vi "MB_TCP_7024_p.vi"(6 "N":i32, 9 "timeouts":T1={"conn_timeout"=1000, "reconn_timeout"=3000, "N attempt max"=3, "t_reset_TTL"=120000, "write_timeout"=10, "read_timeout"=500, "period"=100} {"t_reset_TTL" min=10 max=240000 step=1; "period" min=10 max=100000 step=1; "read_timeout" min=10 max=60000 step=1; "write_timeout" min=1 max=60000 step=1; "N attempt max" min=1 max=5 step=1; "reconn_timeout" min=10 max=240000 step=1; "conn_timeout" min=10 max=240000}, 10 "write enable":bool=TRUE, 11 "stop":bool) -> (0 "error out":errorcluster, 2 "errors":u32, 3 "Z3":u32)   [LabVIEW 2019]
uses:
  NI_modbus_upd/NI_modbus_upd.lvlib
  NI_modbus_upd.llb/MB Modbus Command.ctl
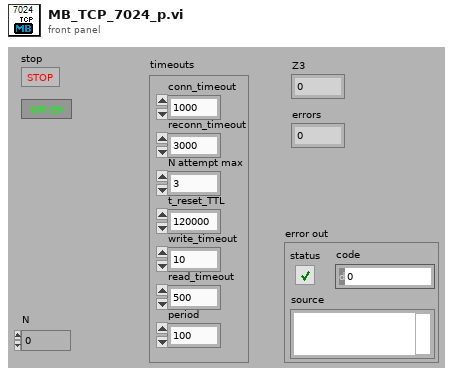
[diagram p1: front panel]
types:
  T1 = cluster{"conn_timeout":i32, "reconn_timeout":u32, "N attempt max":i32, "t_reset_TTL":u32, "write_timeout":i32, "read_timeout":i32, "period":u32}
  T2 = enum16{"Init", "Read", "Read inputs", "Read outputs", "Write", "Write inputs"}
  T3 = enum16{"DI", "DO to write", "DO", "AI", "AO to write", "AO", "DI AI", "DI AO", "DO AI", "DO AO"}
  T4 = enum16{"Start", "Connect", "Write enable", "IP address", "Errors"}
  T5 = typedef "MB Modbus Command.ctl" = cluster{"Function Code":u8, "Starting Address":u16, "Quantity":u16, "Data":u16[], "Discrete":bool[]}
  T6 = cluster{"Transaction ID":u16, "Protocol ID":u16, "Length":u16, "Unit ID":u8}
  T7 = cluster{"Remote IP Address":string, "Remote Port":u16}
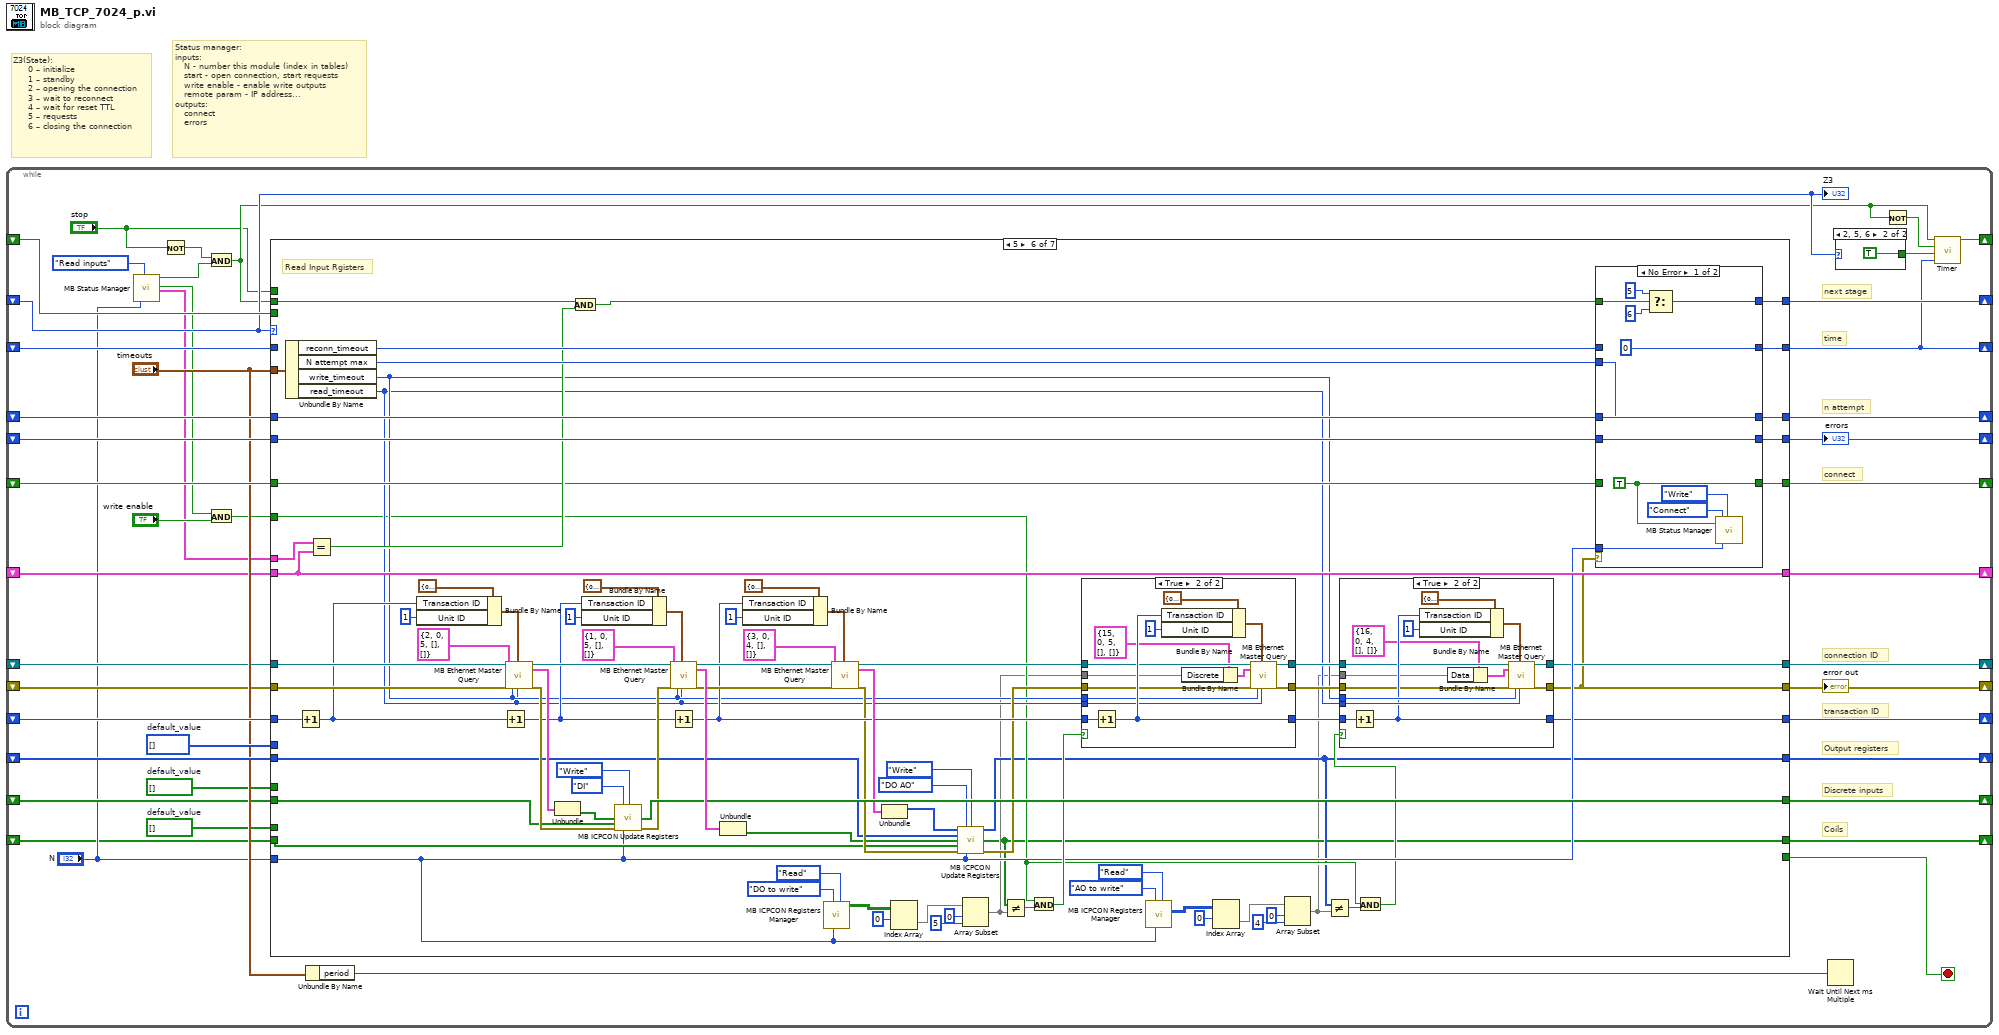
[diagram p0: block diagram]
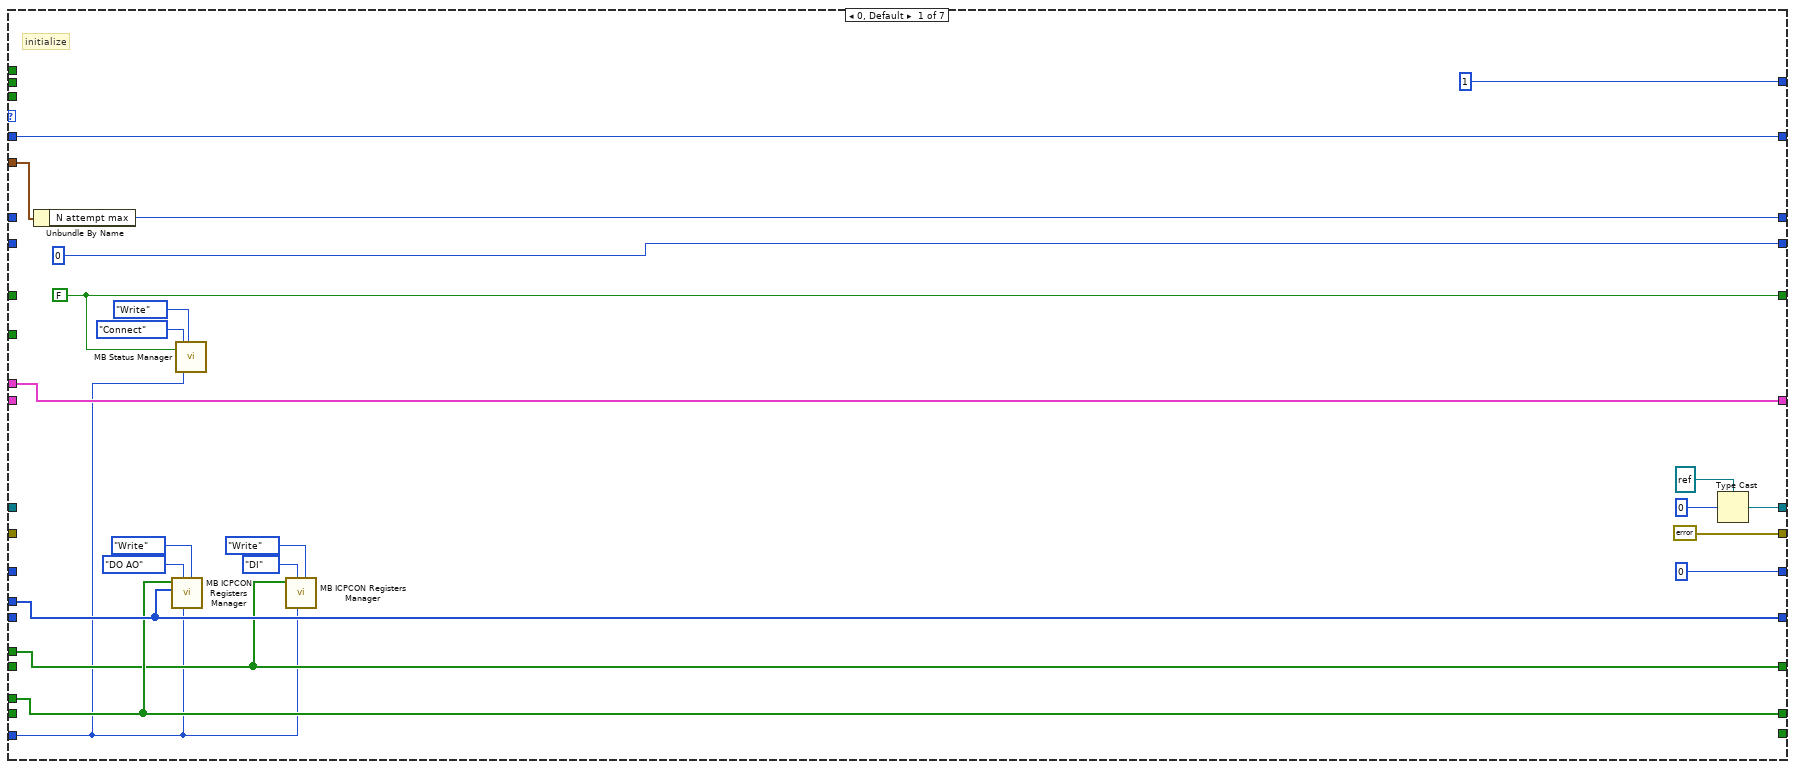
[diagram p2: hidden frame]
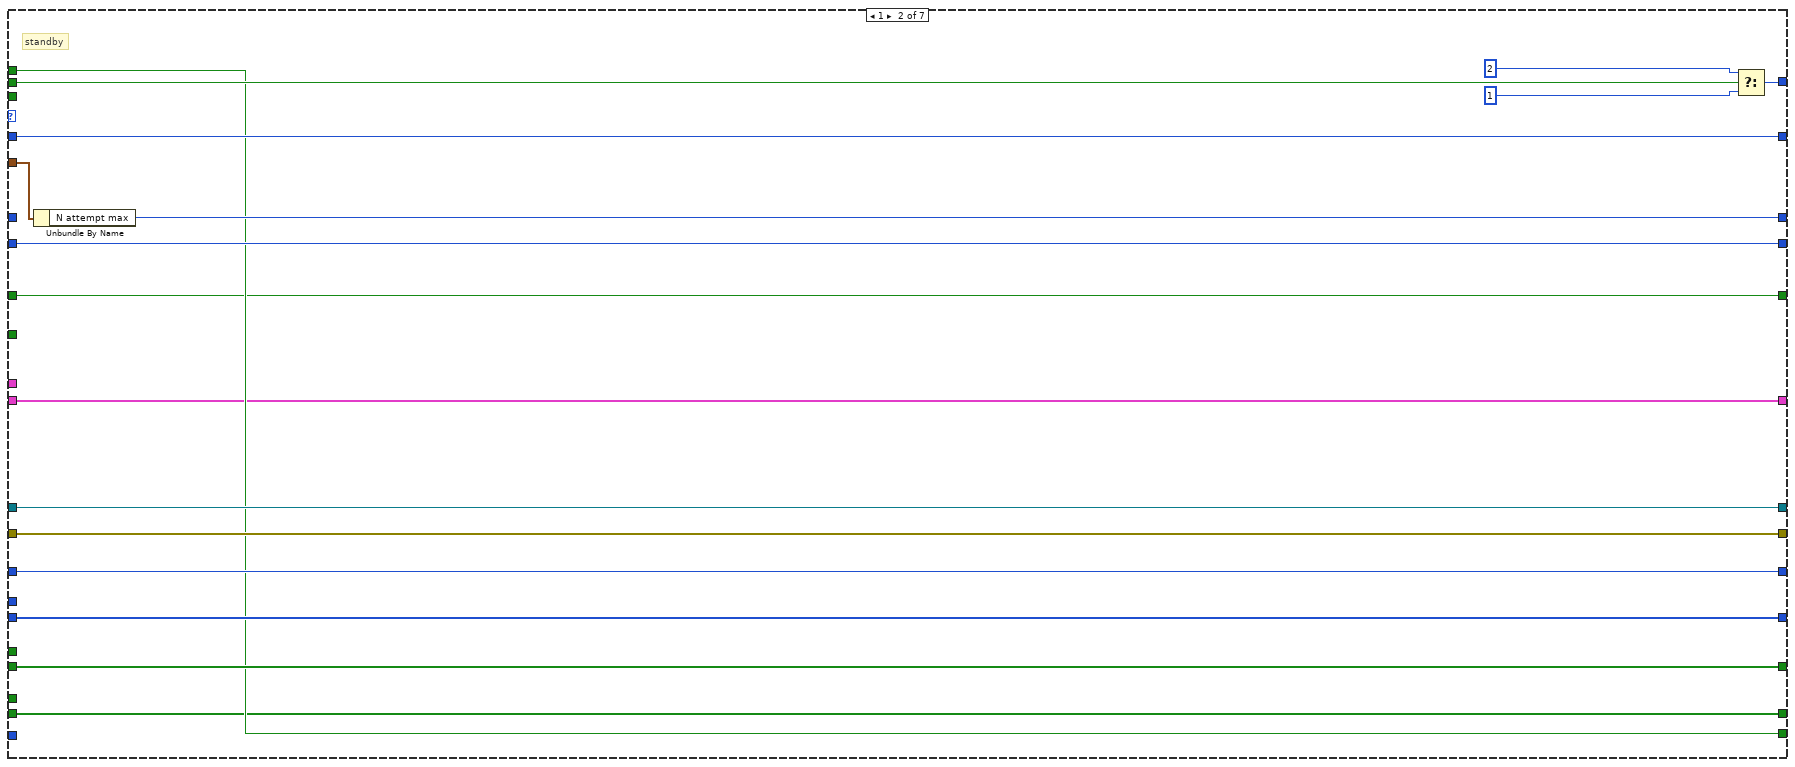
[diagram p3: hidden frame]
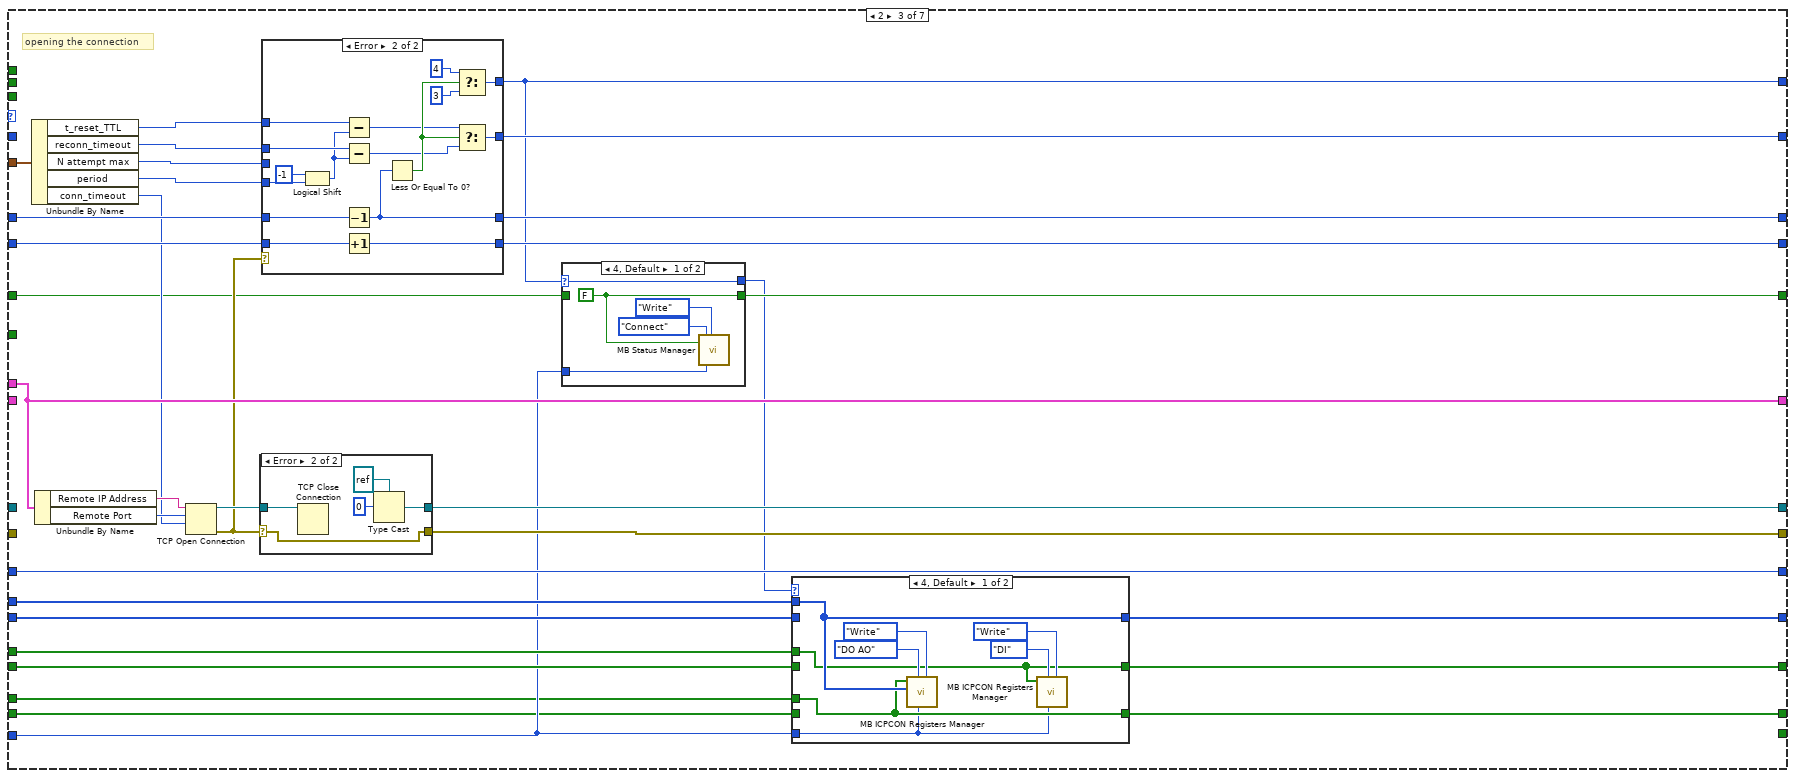
[diagram p4: hidden frame]
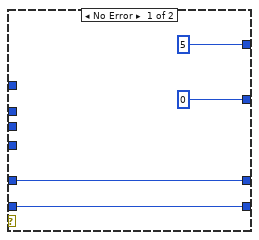
[diagram p8: hidden frame]
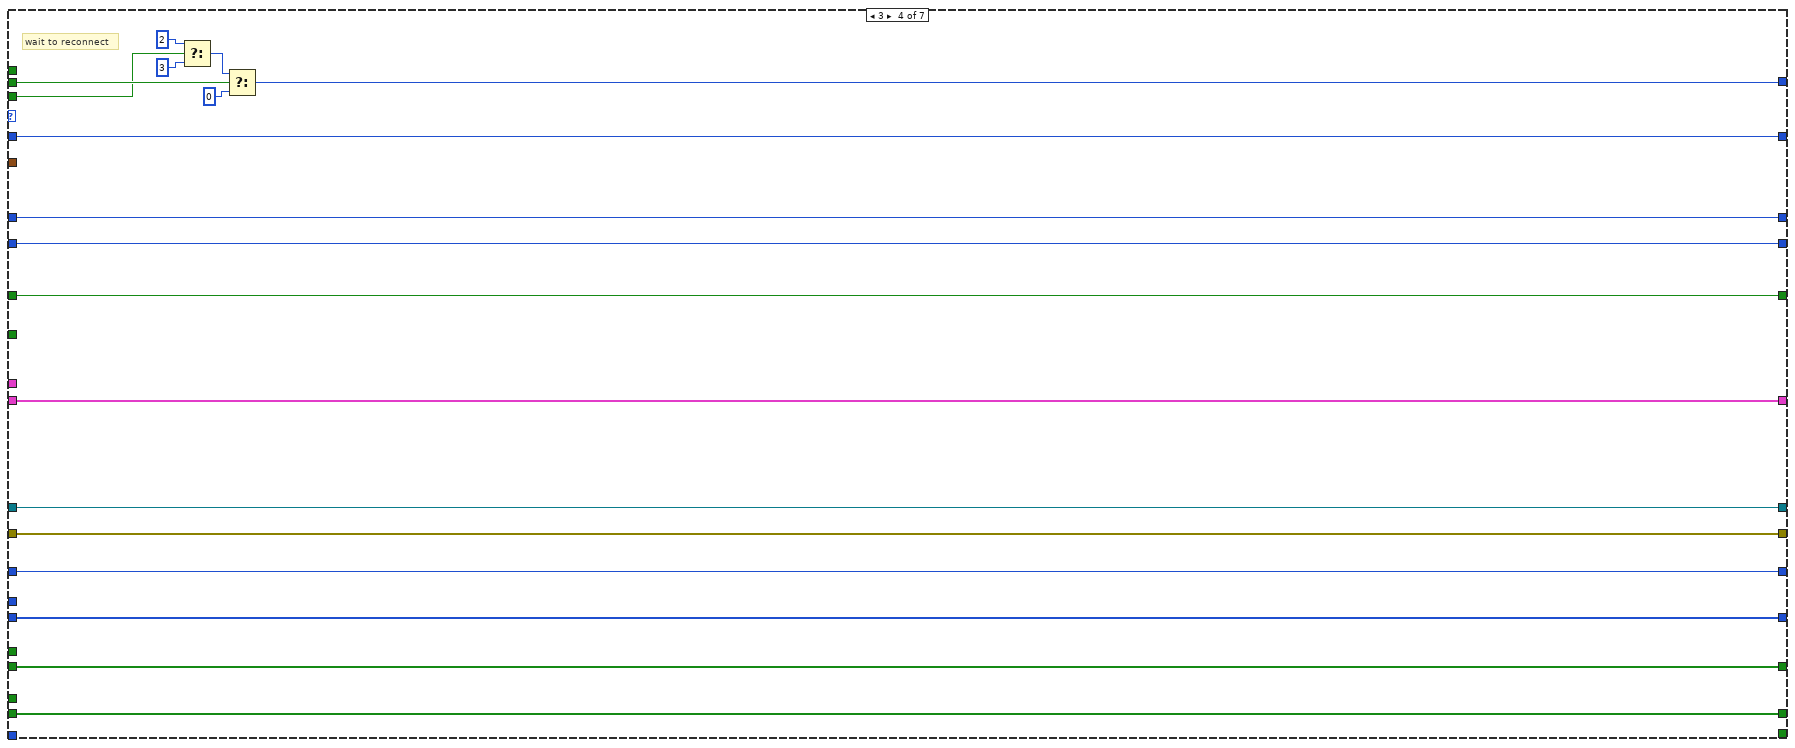
[diagram p9: hidden frame]
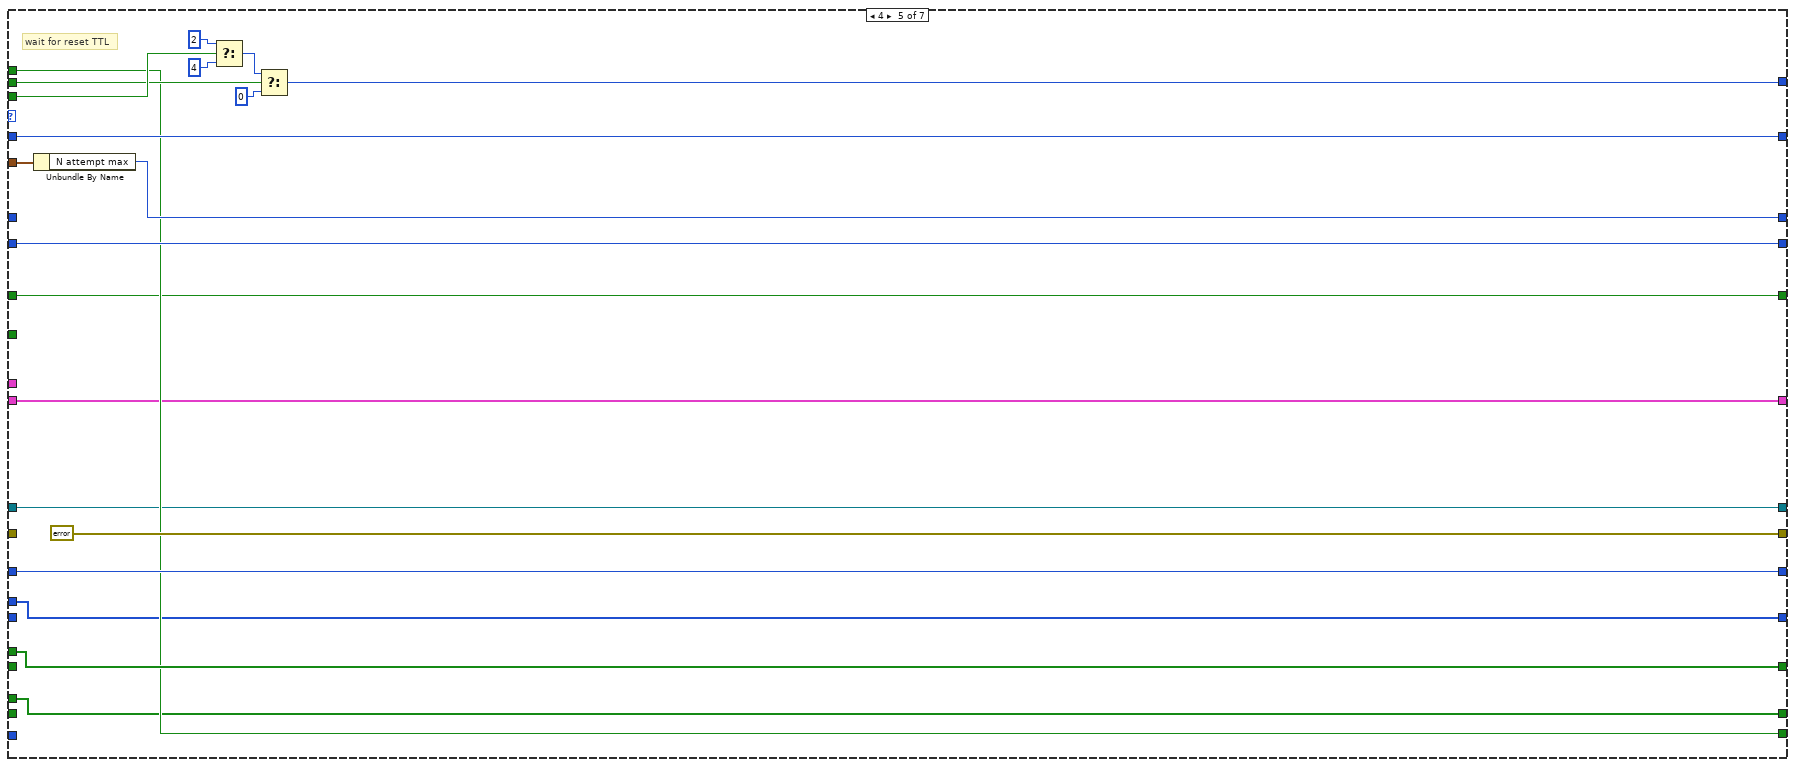
[diagram p10: hidden frame]
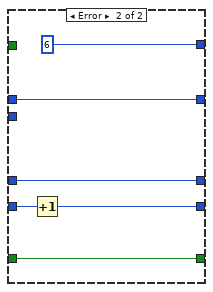
[diagram p13: hidden frame]
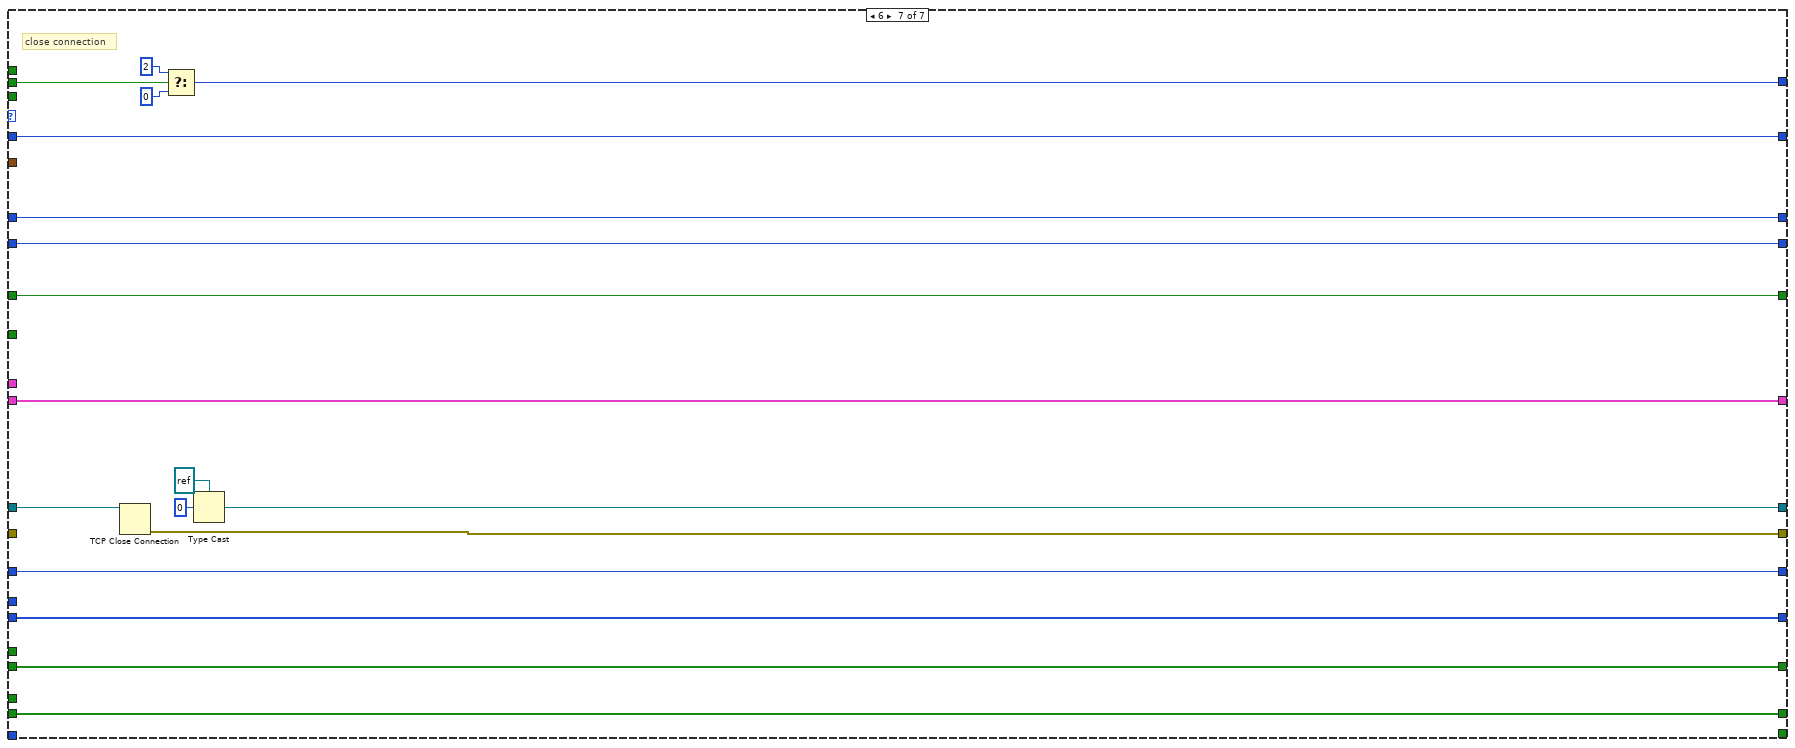
[diagram p14: hidden frame]
diagram:
  # "Status manager:\ninputs:\n   N - number this module (index in tables)\n   start - open connection, start requests\n   write enable - enable write outputs\n   remote param - IP address...\noutputs:\n   connect\n   errors"
  # "Z3(State):\n     0 – initialize \n     1 – standby\n     2 – opening the connection\n     3 – wait to reconnect\n     4 – wait for reset TTL\n     5 – requests\n     6 – closing the connection"
  n1 = while {
    shift-right: [w21] -> _
    shift-left: _ -> [w17]
    shift-right: [w20] -> _
    shift-left: _ -> [w43]
    shift-right: [w42] -> _
    shift-left: _ -> [w40]
    shift-right: [w41] -> _
    shift-left: _ -> [w39]
    shift-right: [w38] -> _
    shift-left: _ -> [w37]
    shift-right: [w36] -> _
    shift-left: _ -> [w22]
    shift-right: [w35] -> _
    shift-left: _ -> [w23]
    shift-right: [w34] -> _
    shift-left: _ -> [w33]
    shift-right: [w32] -> _
    shift-left: _ -> [w31]
    shift-right: [w25] -> _
    shift-left: _ -> [w24]
    shift-right: [w19] -> _
    shift-left: _ -> [w18]
    shift-right: [w10] -> _
    shift-left: _ -> [w9]
    shift-right: [w2] -> _
    shift-left: _ -> [w4]
    stop <- w13 stop-if-true
    w3 = bool[] []  # default_value
    w26 = bool[] []  # default_value
    w30 = u16[] []  # default_value
    # "Coils"
    # "Discrete inputs"
    # "Output registers"
    # "connect"
    # "connection ID"
    # "transaction ID"
    # "n attempt"
    # "time"
    # "next stage"
    n2 = call "MB Status Manager.vi"("N"="N", "Function"=T2."Read inputs") -> ("start"=w8:bool, "write enable"=w7:bool, "Remote Param"=w6:T7)  [unwired: 12 in, 3 out]
    n3 = Not(x="stop") -> (.not. x?=w15:bool)
    n4 = And(x=w15, y=w8) -> (x .and. y?=w16:bool)
    n5 = And(x=w7, y="write enable") -> (x .and. y?=w12:bool)
    n6 = case shown="5" w17 {
      tunnel: [w64 w74 w94 w177 w184 w213 w353] -> w36
      tunnel: [errorcluster {"status"=FALSE, "code"=0, "source"=""} ("error out") w73 w92 w176 errorcluster {"status"=FALSE, "code"=0, "source"=""} ("error out") w211 w354] -> w35
      tunnel: w22 -> [_ w74 _ w177 w184 w277 w350]
      tunnel: w23 -> [_ w73 _ w176 _ w276 _]
      tunnel: [w53 w69 w90 w165 w183 w264 w341] -> w38
      tunnel: w37 -> [_ w69 w91 w165 w183 w265 w341]
      tunnel: w6 -> [w56 _ w97 _ _ w271 _]
      tunnel: [w52 w75 w102 w164 w180 w203 w340] -> w32
      tunnel: w31 -> [_ w75 w103 w164 _ w225 w340]
      tunnel: w33 -> [_ w83 w116 w179 w199 w286 w355]
      tunnel: [u16 0 ("x") w83 w116 w179 w199 w209 w355] -> w34
      tunnel: [w58 w79 w111 w178 w195 w284 w347] -> w42
      tunnel: w40 -> [_ _ w112 w178 _ w284 w347]
      tunnel: [u32 0 ("N attempt max") w82 w114 w175 w198 w283 w352] -> w41
      tunnel: w39 -> [_ w82 w115 w175 w198 w282 w352]
      tunnel: [w60 w81 w108 w174 w197 w279 w351] -> w20
      tunnel: w43 -> [w60 w81 _ w174 w197 _ w351]
      tunnel: "timeouts" -> [w59 w80 w113 _ w196 w285 _]
      tunnel: w16 -> [_ w71 _ w170 w186 w270 w348]
      tunnel: [u32 1 w76 w88 w166 w190 w278 w342] -> w21
      tunnel: w18 -> [_ _ _ w168 w189 _ _]
      tunnel: w30 -> [w52 _ w101 _ w180 _ _]
      tunnel: w26 -> [w47 _ w98 _ w187 _ _]
      tunnel: [w47 w72 w99 w167 w187 w254 w345] -> w25
      tunnel: w24 -> [_ w72 w100 w167 _ w227 w345]
      tunnel: "N" -> [w46 _ w89 _ _ w216 _]
      tunnel: "stop" -> [_ w70 _ _ w185 _ _]
      tunnel: [_ w70 _ _ w185 _ _] -> w13
      tunnel: w12 -> [_ _ _ _ _ w205 _]
      tunnel: [w56 w68 w97 w163 w182 w268 w339] -> w10
      tunnel: w9 -> [_ w68 _ w163 w182 w268 w339]
      tunnel: w3 -> [w50 _ w86 _ w181 _ _]
      tunnel: w4 -> [_ w67 w85 w162 _ w223 w338]
      tunnel: [w50 w67 w84 w162 w181 w201 w338] -> w2
      frame 0, Default {
        w53 = FALSE ("connect")
        # "initialize"
        n7 = Unbundle By Name(w59) -> ("N attempt max"=w58:i32)
        n8 = call "MB ICPCON Registers Manager.vi"("Function"=enum16{"Init", "Read", "Write", "Read All"}."Write", "N"=w46, "Table"=T3."DO AO", "Registers In"=w52, "Discrete in"=w50) -> ()  [unwired: 4 in, 3 out]
        n9 = call "MB Status Manager.vi"("connect in"=w53, "Table"=T4."Connect", "N"=w46, "Function"=T2."Write") -> ()  [unwired: 10 in, 6 out]
        n10 = call "MB ICPCON Registers Manager.vi"("Function"=enum16{"Init", "Read", "Write", "Read All"}."Write", "N"=w46, "Table"=T3."DI", "Discrete in"=w47) -> ()  [unwired: 5 in, 3 out]
        n11 = Type Cast(type=refnum<k5> refnum ("connection ID"), x=u32 0) -> (*(type *) &x=w64:refnum<k5>)
      }
      frame 1 {
        # "standby"
        n12 = Unbundle By Name(w80) -> ("N attempt max"=w79:i32)
        n13 = Select(t=u32 2, s=w71, f=u32 1) -> (s? t:f=w76:u32)
      }
      frame 2 {
        # "opening the connection"
        n14 = Unbundle By Name(w113) -> ("t_reset_TTL"=w107:u32, "reconn_timeout"=w109:u32, "N attempt max"=w110:i32, "period"=w104:u32, "conn_timeout"=w96:i32)
        n15 = Unbundle By Name(w97) -> ("Remote IP Address"=w106:string, "Remote Port"=w105:u16)
        n16 = TCP Open Connection(address=w106, remote port or service name=w105, timeout ms (60000)=w96) -> (connection ID=w95:refnum<k5>, error out=w93:errorcluster)  [unwired: 2 in]
        n17 = case shown="Error" w93 {
          selector: w93 -> [w124 w126]
          tunnel: w95 -> [w125 w129]
          tunnel: [w125 w128] -> w94
          tunnel: [w124 w126] -> w92
          frame No Error {
          }
          frame Error {
            n18 = TCP Close Connection(connection ID=w129) -> ()  [unwired: 2 in, 2 out]
            n19 = Type Cast(type=refnum<k5> refnum ("connection ID"), x=u32 0) -> (*(type *) &x=w128:refnum<k5>)
          }
        }
        n20 = case shown="Error" w93 {
          tunnel: w115 -> [w145 w161]
          tunnel: [w145 w160] -> w114
          tunnel: w112 -> [w144 w159]
          tunnel: [w144 w158] -> w111
          tunnel: w110 -> [_ _]
          tunnel: [u32 5 w155] -> w88
          tunnel: w109 -> [_ w154]
          tunnel: [u32 0 w153] -> w108
          tunnel: w107 -> [_ w150]
          tunnel: w104 -> [_ w148]
          frame No Error {
          }
          frame Error {
            n21 = Logical Shift(y=i16 -1, x=w148) -> (x << y=w146:u32)
            n22 = Subtract(x=w150, y=w146) -> (x-y=w149:u32)
            n23 = Subtract(x=w154, y=w146) -> (x-y=w151:u32)
            n24 = Decrement(x=w159) -> (x-1=w158:i32)
            n25 = Increment(x=w161) -> (x+1=w160:u32)
            n26 = Less Or Equal To 0?(x=w158) -> (x <= 0?=w152:bool)
            n27 = Select(t=u32 4, s=w152, f=u32 3) -> (s? t:f=w155:u32)
            n28 = Select(t=w149, s=w152, f=w151) -> (s? t:f=w153:u32)
          }
        }
        n29 = case shown="4, Default" w88 {
          selector: w88 -> [w118 w122]
          tunnel: w89 -> [w119 _]
          tunnel: [w120 w123] -> w90
          tunnel: w91 -> [_ w123]
          tunnel: [w118 w122] -> w87
          frame 4, Default {
            w120 = FALSE ("f")
            n30 = call "MB Status Manager.vi"("connect in"=w120, "Table"=T4."Connect", "N"=w119, "Function"=T2."Write") -> ()  [unwired: 10 in, 6 out]
          }
          frame 3, 5 {
          }
        }
        n31 = case shown="4, Default" w87 {
          tunnel: w89 -> [w132 _]
          tunnel: [w136 w141] -> w102
          tunnel: w103 -> [_ w141]
          tunnel: w101 -> [w136 _]
          tunnel: w100 -> [_ w140]
          tunnel: [w131 w140] -> w99
          tunnel: w98 -> [w131 _]
          tunnel: w86 -> [w135 _]
          tunnel: [w135 w139] -> w84
          tunnel: w85 -> [_ w139]
          frame 4, Default {
            n32 = call "MB ICPCON Registers Manager.vi"("Function"=enum16{"Init", "Read", "Write", "Read All"}."Write", "N"=w132, "Table"=T3."DO AO", "Registers In"=w136, "Discrete in"=w135) -> ()  [unwired: 4 in, 3 out]
            n33 = call "MB ICPCON Registers Manager.vi"("Function"=enum16{"Init", "Read", "Write", "Read All"}."Write", "N"=w132, "Table"=T3."DI", "Discrete in"=w131) -> ()  [unwired: 5 in, 3 out]
          }
          frame 3, 5 {
          }
        }
      }
      frame 3 {
        # "wait to reconnect"
        n34 = Select(t=u32 2, s=w168, f=u32 3) -> (s? t:f=w169:u32)
        n35 = Select(t=w169, s=w170, f=u32 0) -> (s? t:f=w166:u32)
      }
      frame 4 {
        # "wait for reset TTL"
        n36 = Unbundle By Name(w196) -> ("N attempt max"=w195:i32)
        n37 = Select(t=u32 2, s=w189, f=u32 4) -> (s? t:f=w191:u32)
        n38 = Select(t=w191, s=w186, f=u32 0) -> (s? t:f=w190:u32)
      }
      frame 5 {
        # "Read Input Rgisters"
        n39 = Unbundle By Name(w285) -> ("reconn_timeout"=w280:u32, "N attempt max"=w281:i32, "write_timeout"=w208:i32, "read_timeout"=w207:i32)
        n40 = Increment(x=w286) -> (x+1=w258:u16)
        n41 = Equal?(x=w271, y=w268) -> (x = y?=w267:bool)
        n42 = Bundle By Name(cluster=T6 {"Transaction ID"=0, "Protocol ID"=0, "Length"=0, "Unit ID"=0} ("MBAP Header"), "Transaction ID"=w258, "Unit ID"=u8 1) -> (w272:T6)
        n43 = Increment(x=w258) -> (x+1=w242:u16)
        n44 = call "MB Ethernet Master Query.vi"("TCP Connection Refnum in"=w277, "Modbus Command"=T5 {"Function Code"=2, "Starting Address"=0, "Quantity"=5, "Data"=[], "Discrete"=[]}, "error in (no error)"=w276, "Write Timeout"=w208, "MBAP Header"=w272, "Read Timeout"=w207) -> ("TCP Connection Refnum (dup)"=w252:refnum<k5>, "Registers"=w275:cluster{"Registers":u16[], "Discrete":bool[]}, "error out"=w251:errorcluster)  [unwired: 9 in, 2 out]
        n45 = Unbundle(w275) -> ("Discrete"=w228:bool[])  [unwired: 1 out]
        n46 = And(x=w270, y=w267) -> (x .and. y?=w269:bool)
        n47 = Bundle By Name(cluster=T6 {"Transaction ID"=0, "Protocol ID"=0, "Length"=0, "Unit ID"=0} ("MBAP Header"), "Transaction ID"=w242, "Unit ID"=u8 1) -> (w261:T6)
        n48 = call "MB ICPCON Update Registers.vi"("Table"=T3."DI", "Function"=enum16{"Init", "Read", "Write", "Read All"}."Write", "Discrete in"=w228, "Default Discrete in"=w227, "error in (no error)"=w251, "N"=w216) -> ("Discretes"=w254:bool[], "error out"=w250:errorcluster)  [unwired: 7 in, 1 out]
        n49 = call "MB Ethernet Master Query.vi"("TCP Connection Refnum in"=w252, "Modbus Command"=T5 {"Function Code"=1, "Starting Address"=0, "Quantity"=5, "Data"=[], "Discrete"=[]} ("MODBUS Command"), "error in (no error)"=w250, "Write Timeout"=w208, "MBAP Header"=w261, "Read Timeout"=w207) -> ("TCP Connection Refnum (dup)"=w244:refnum<k5>, "Registers"=w256:cluster{"Registers":u16[], "Discrete":bool[]}, "error out"=w241:errorcluster)  [unwired: 9 in, 2 out]
        n50 = Increment(x=w242) -> (x+1=w240:u16)
        n51 = Unbundle(w256) -> ("Discrete"=w224:bool[])  [unwired: 1 out]
        n52 = Bundle By Name(cluster=T6 {"Transaction ID"=0, "Protocol ID"=0, "Length"=0, "Unit ID"=0} ("MBAP Header"), "Transaction ID"=w240, "Unit ID"=u8 1) -> (w245:T6)
        n53 = call "MB ICPCON Registers Manager.vi"("Function"=enum16{"Init", "Read", "Write", "Read All"}."Read", "N"=w216, "Table"=T3."DO to write") -> ("Discretes"=w235:bool[][])  [unwired: 6 in, 2 out]
        n54 = call "MB Ethernet Master Query.vi"("TCP Connection Refnum in"=w244, "Modbus Command"=T5 {"Function Code"=3, "Starting Address"=0, "Quantity"=4, "Data"=[], "Discrete"=[]} ("MODBUS Command"), "error in (no error)"=w241, "MBAP Header"=w245) -> ("TCP Connection Refnum (dup)"=w243:refnum<k5>, "Registers"=w249:cluster{"Registers":u16[], "Discrete":bool[]}, "error out"=w230:errorcluster)  [unwired: 11 in, 2 out]
        n55 = Unbundle(w249) -> ("Registers"=w226:u16[])  [unwired: 1 out]
        n56 = Index Array(array=w235, index (row)=0) -> (element=w233:bool[])  [unwired: 1 in]
        n57 = call "MB ICPCON Update Registers.vi"("Registers In"=w226, "Table"=T3."DO AO", "Function"=enum16{"Init", "Read", "Write", "Read All"}."Write", "Default Registers In"=w225, "Discrete in"=w224, "Default Discrete in"=w223, "error in (no error)"=w230, "N"=w216) -> ("Registers"=w203:u16[], "Discretes"=w201:bool[], "error out"=w229:errorcluster)  [unwired: 5 in]
        n58 = Array Subset(array=w233, index=0, length=5) -> (w202:bool[])
        n59 = Not Equal?(x=w201, y=w202) -> (x != y?=w255:bool)
        n60 = And(x=w205, y=w255) -> (x .and. y?=w253:bool)
        n61 = case shown="True" w253 {
          tunnel: w207 -> [_ w311]
          tunnel: w208 -> [_ w310]
          tunnel: w240 -> [w305 w318]
          tunnel: [w305 w317] -> w210
          tunnel: w229 -> [w304 w315]
          tunnel: [w304 w314] -> w212
          tunnel: w243 -> [w306 w313]
          tunnel: [w306 w312] -> w214
          tunnel: w202 -> [_ w307]
          frame False {
          }
          frame True {
            n62 = Increment(x=w318) -> (x+1=w317:u16)
            n63 = Bundle By Name(cluster=T6 {"Transaction ID"=0, "Protocol ID"=0, "Length"=0, "Unit ID"=0} ("MBAP Header"), "Transaction ID"=w317, "Unit ID"=u8 1) -> (w319:T6)
            n64 = Bundle By Name(cluster=T5 {"Function Code"=15, "Starting Address"=0, "Quantity"=5, "Data"=[], "Discrete"=[]} ("MODBUS Command"), "Discrete"=w307) -> (w308:T5)
            n65 = call "MB Ethernet Master Query.vi"("TCP Connection Refnum in"=w313, "Modbus Command"=w308, "error in (no error)"=w315, "Write Timeout"=w310, "MBAP Header"=w319, "Read Timeout"=w311) -> ("TCP Connection Refnum (dup)"=w312:refnum<k5>, "error out"=w314:errorcluster)  [unwired: 9 in, 3 out]
          }
        }
        n66 = call "MB ICPCON Registers Manager.vi"("Function"=enum16{"Init", "Read", "Write", "Read All"}."Read", "N"=w216, "Table"=T3."AO to write") -> ("Registers"=w215:u16[][])  [unwired: 6 in, 2 out]
        n67 = Index Array(array=w215, index (row)=0) -> (element=w222:u16[])  [unwired: 1 in]
        n68 = Array Subset(array=w222, index=0, length=4) -> (w200:u16[])
        n69 = Not Equal?(x=w203, y=w200) -> (x != y?=w206:bool)
        n70 = And(x=w205, y=w206) -> (x .and. y?=w204:bool)
        n71 = case shown="True" w204 {
          tunnel: w207 -> [_ w301]
          tunnel: w208 -> [_ w300]
          tunnel: w210 -> [w288 w299]
          tunnel: [w288 w298] -> w209
          tunnel: w212 -> [w287 w296]
          tunnel: [w287 w295] -> w211
          tunnel: w214 -> [w289 w294]
          tunnel: [w289 w293] -> w213
          tunnel: w200 -> [_ w290]
          frame False {
          }
          frame True {
            n72 = Increment(x=w299) -> (x+1=w298:u16)
            n73 = Bundle By Name(cluster=T6 {"Transaction ID"=0, "Protocol ID"=0, "Length"=0, "Unit ID"=0} ("MBAP Header"), "Transaction ID"=w298, "Unit ID"=u8 1) -> (w302:T6)
            n74 = Bundle By Name(cluster=T5 {"Function Code"=16, "Starting Address"=0, "Quantity"=4, "Data"=[], "Discrete"=[]} ("MODBUS Command"), "Data"=w290) -> (w291:T5)
            n75 = call "MB Ethernet Master Query.vi"("TCP Connection Refnum in"=w294, "Modbus Command"=w291, "error in (no error)"=w296, "Write Timeout"=w300, "MBAP Header"=w302, "Read Timeout"=w301) -> ("TCP Connection Refnum (dup)"=w293:refnum<k5>, "error out"=w295:errorcluster)  [unwired: 9 in, 3 out]
          }
        }
        n76 = case shown="No Error" w211 {
          tunnel: w282 -> [w325 w337]
          tunnel: [w325 w336] -> w283
          tunnel: [w327 u32 6] -> w278
          tunnel: w284 -> [_ w334]
          tunnel: w281 -> [w331 _]
          tunnel: [w331 w334] -> _
          tunnel: w280 -> [_ w333]
          tunnel: [u32 0 w333] -> w279
          tunnel: w269 -> [w326 _]
          tunnel: w265 -> [_ w332]
          tunnel: [w323 w332] -> w264
          tunnel: w216 -> [w322 _]
          frame No Error {
            w323 = TRUE ("f")
            n77 = Select(t=u32 5, s=w326, f=u32 6) -> (s? t:f=w327:u32)
            n78 = call "MB Status Manager.vi"("connect in"=w323, "Table"=T4."Connect", "N"=w322, "Function"=T2."Write") -> ()  [unwired: 10 in, 6 out]
          }
          frame Error {
            n79 = Increment(x=w337) -> (x+1=w336:u32)
          }
        }
      }
      frame 6 {
        # "close connection"
        n80 = TCP Close Connection(connection ID=w350) -> (error out=w354:errorcluster)  [unwired: 2 in, 1 out]
        n81 = Select(t=u32 2, s=w348, f=u32 0) -> (s? t:f=w342:u32)
        n82 = Type Cast(type=refnum<k5> refnum ("connection ID"), x=u32 0) -> (*(type *) &x=w353:refnum<k5>)
      }
    }
    "error out" <- w35
    "errors" <- w41
    n83 = Unbundle By Name("timeouts") -> ("period"=w28:u32)
    n84 = Wait Until Next ms Multiple(millisecond multiple=w28) -> ()  [unwired: 1 out]
    n85 = case shown="2, 5, 6" w17 {
      tunnel: [_ TRUE] -> w27
      frame 0, Default {
      }
      frame 2, 5, 6 {
      }
    }
    n86 = Not(x=w16) -> (.not. x?=w44:bool)
    n87 = call "Timer.vi"("ms"=w20, "Load (F)"=w27, "Reset (F)"=w44, "Start (T)"=w16) -> ("End"=w19:bool)  [unwired: 5 in, 1 out]
    "Z3" <- w17
  }
